vi "Manual Query.vi"(8 "error in (no error)":errorcluster, 9 "Timeout (1s)":dbl[unit]=1.0, 10 "Command":string, 11 "VISA resource name":refnum<visa-resource-name>) -> (0 "error out":errorcluster, 2 "Response":string, 3 "VISA resource name out":refnum<visa-resource-name>)   [LabVIEW 2013, in "HadCon.lvlib"]
doc: "Send a text command and read response.."
uses:
  <instrlib>/HadCon/HadCon.lvlib
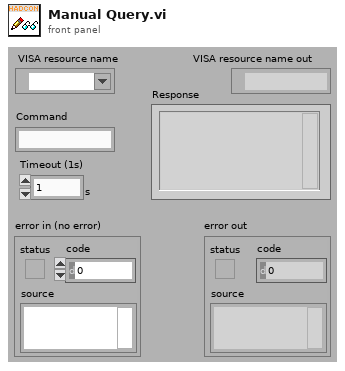
[diagram p1: front panel]
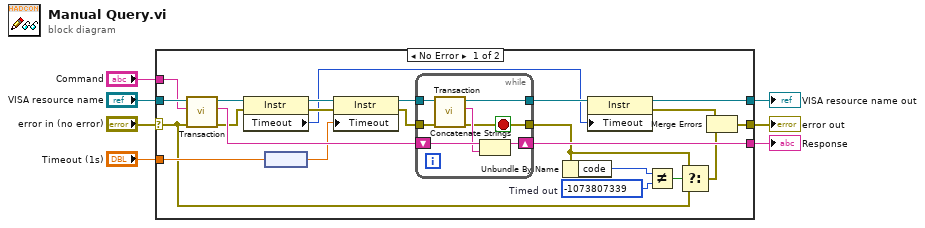
[diagram p0: block diagram]
diagram:
  n1 = case shown="No Error" "error in (no error)" {
    selector: "error in (no error)" -> [w10 w38]
    tunnel: [w8 w39] -> w7
    tunnel: "VISA resource name" -> [w30 w39]
    tunnel: [w9 w38] -> w5
    tunnel: [w27 _] -> w4
    tunnel: "Command" -> [w13 _]
    tunnel: "Timeout (1s)" -> [w12 _]
    frame No Error {
      w24 = -1073807339  # Timed out
      n2 = call <instrlib>:"Transaction.vi"("Error In"=w10, "Command"=w13, "VISA resource name"=w30) -> ("Error Out"=w20:errorcluster, "Response"=w28:string, "VISA resource name out"=w29:refnum<visa-resource-name>)  [unwired: 6 in]
      n3 = property class="Instr"(reference=w29, error in=w20) -> (reference out=w21:refnum<visa-resource-name>, error out=w18:errorcluster, "Timeout"=w16:u32)
      n4 = node(w12) -> (w11:dbl)
      n5 = property class="Instr"(reference=w21, error in=w18, "Timeout"=w11) -> (reference out=w19:refnum<visa-resource-name>, error out=w17:errorcluster)
      n6 = while {
        tunnel: w19 -> [w37]
        tunnel: w17 -> [w36]
        shift-right: [w33] -> w27
        shift-left: w28 -> [w35]
        tunnel: [w32] -> w26
        tunnel: [w31] -> w22
        stop <- w31 stop-if-true
        n7 = call <instrlib>:"Transaction.vi"("Error In"=w36, "VISA resource name"=w37) -> ("Error Out"=w31:errorcluster, "Response"=w34:string, "VISA resource name out"=w32:refnum<visa-resource-name>)  [unwired: 7 in]
        n8 = Concatenate Strings(w35, w34) -> (w33:string)
      }
      n9 = Unbundle By Name(w22) -> ("code"=w25:i32)
      n10 = property class="Instr"(reference=w26, "Timeout"=w16) -> (reference out=w8:refnum<visa-resource-name>, error out=w15:errorcluster)  [unwired: 1 in]
      n11 = Not Equal?(x=w25, y=w24) -> (x != y?=w23:bool)
      n12 = Select(t=w22, s=w23, f=w10) -> (s? t:f=w14:errorcluster)
      n13 = Merge Errors(w15, w14) -> (w9:errorcluster)
    }
    frame Error {
    }
  }
  "VISA resource name out" <- w7
  "error out" <- w5
  "Response" <- w4
